vi "SoftReset.vi"(8 "error in (no error)":errorcluster, 11 "BME680 in":refnum<class "BME680.lvclass">) -> (0 "error out":errorcluster, 3 "BME680 out":refnum<class "BME680.lvclass">)   [LabVIEW 2022 SP3, in "BME680.lvlib" / "BME680.lvclass"]
uses:
  BME680.lvclass
  BME680.lvclass/BME680.ctl
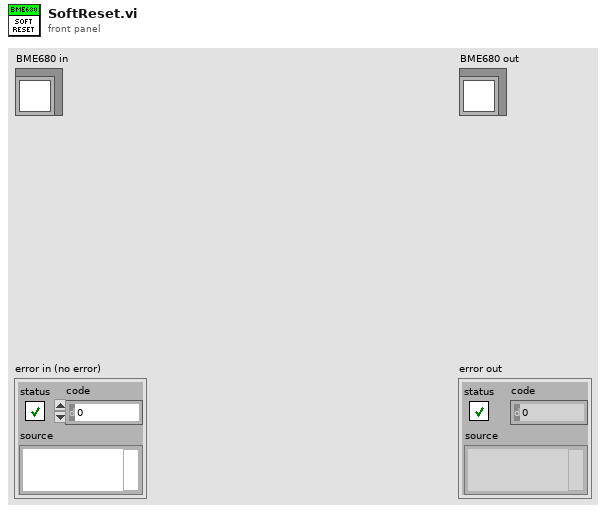
[diagram p1: front panel]
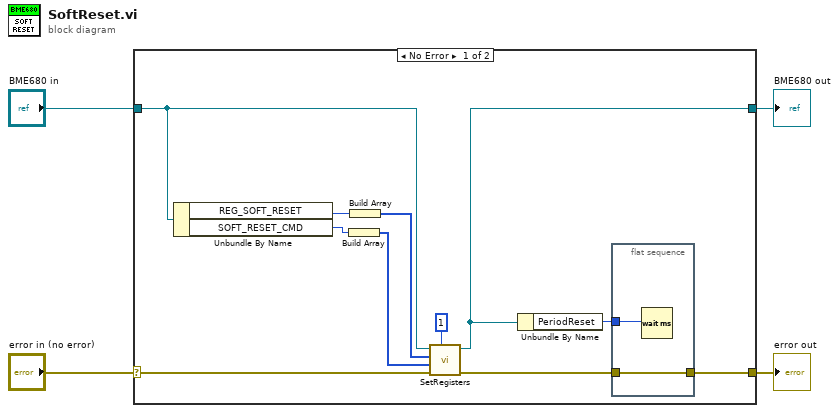
[diagram p0: block diagram]
diagram:
  n1 = case shown="No Error" "error in (no error)" {
    selector: "error in (no error)" -> [w15 w19]
    tunnel: [w7 w19] -> w3
    tunnel: [w6 w18] -> w1
    tunnel: "BME680 in" -> [w13 w18]
    frame No Error {
      n2 = Unbundle By Name(w13) -> ("REG_SOFT_RESET"=w11:u8, "SOFT_RESET_CMD"=w12:u8)
      n3 = Build Array(w12) -> (w10:u8[])
      n4 = Build Array(w11) -> (w9:u8[])
      n5 = call-dynamic "SetRegisters.vi"("Lenght"=1, "error in (no error)"=w15, "Register Data"=w10, "Register Addres"=w9, "BME680 in"=w13) -> ("error out"=w8:errorcluster, "BME680 out"=w6:refnum<class "BME680.lvclass">)  [unwired: 5 in]
      n6 = Unbundle By Name(w6) -> ("PeriodReset"=w5:u32)
      n7 = flat-sequence {
        tunnel: [w17] -> w7
        tunnel: w8 -> [w17]
        tunnel: w5 -> [w16]
        frame #0 {
          n8 = Wait (ms)(milliseconds to wait=w16) -> ()  [unwired: 1 out]
        }
      }
    }
    frame Error {
    }
  }
  "error out" <- w3
  "BME680 out" <- w1
